vi "Set Tray Icon (file).vi"(0 "NotifyIcon in":refnum<class "NotifyIcon.lvclass">, 7 "Image file":path, 11 "error in (no error)":errorcluster) -> (4 "NotifyIcon out":refnum<class "NotifyIcon.lvclass">, 15 "error out":errorcluster)   [LabVIEW 2016, in "NotifyIcon.lvclass"]
doc: "This VI is used to set the icon that is associated with the context menu and shown in the notification area.\nThis VI loads a specified BMP, GIF, JPG, PNG, TIFF or ICO file and uses the content as the icon. The loaded file image is automatically resized to fit the notification area.\n\n\nStinus Olsen\nCIM Industrial Systems A/S\n22. Feb. 2011 15:06\nmailto: seo@cim.as"
uses:
  NotifyIcon.lvclass
  System.Drawing
panel:
  # "This VI belongs to the NotifyIcon Toolset. \nA toolset that makes it easy to create, control and manipulate a notification icon in the notification area of the Windows taskbar.\nThe toolset requires Microsoft .NET framework 2.0\n\n\nNOTICE -- YOU MUST LEAVE THIS NOTICE IN PLACE.  PER THE TERMS OF THE LICENSE BELOW, YOU MAY SUBLICENSE THIS SOFTWARE \nIN ANY WAY THAT DOES NOT CONFLICT WITH THIS LICENSE.\n\n### BSD License (http://www.opensource.org/licenses/bsd-license.php) Begin ###\n \nCopyright (c) 2011, Stinus Olsen <seo@cim.as>\n\nAll rights reserved.\n\nRedistribution and use in source and binary forms, with or without modification, are permitted provided that the following conditions are met:\n\n    * Redistributions of source code must retain the above copyright notice, this list of conditions and the following disclaimer.\n    * Redistributions in binary form must reproduce the above copyright notice, this list of conditions and the following disclaimer in the \n       documentation and/or other materials provided with the distribution.\n    * Neither the name of CIM Industrial Systems nor the names of its contributors may be used to endorse or promote products derived \n       from this software without specific prior written permission.\n\nTHIS SOFTWARE IS PROVIDED BY THE COPYRIGHT HOLDERS AND CONTRIBUTORS \"AS IS\" AND ANY EXPRESS OR IMPLIED WARRANTIES, \nINCLUDING, BUT NOT LIMITED TO, THE IMPLIED WARRANTIES OF MERCHANTABILITY AND FITNESS FOR A PARTICULAR PURPOSE ARE \nDISCLAIMED. IN NO EVENT SHALL THE COPYRIGHT OWNER OR CONTRIBUTORS BE LIABLE FOR ANY DIRECT, INDIRECT, INCIDENTAL,\n SPECIAL, EXEMPLARY, OR CONSEQUENTIAL DAMAGES (INCLUDING, BUT NOT LIMITED TO, PROCUREMENT OF SUBSTITUTE GOODS OR \nSERVICES; LOSS OF USE, DATA, OR PROFITS; OR BUSINESS INTERRUPTION) HOWEVER CAUSED AND ON ANY THEORY OF LIABILITY, \nWHETHER IN CONTRACT, STRICT LIABILITY, OR TORT (INCLUDING NEGLIGENCE OR OTHERWISE) ARISING IN ANY WAY OUT OF THE USE \nOF THIS SOFTWARE, EVEN IF ADVISED OF THE POSSIBILITY OF SUCH DAMAGE.\n\n### BSD License End ###"
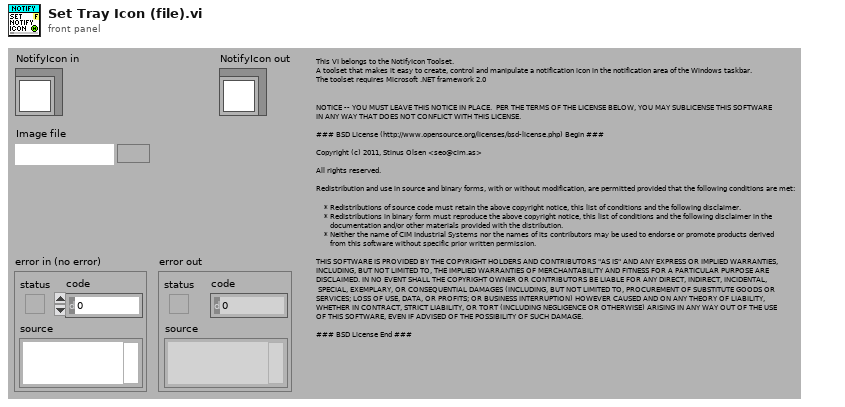
[diagram p1: front panel]
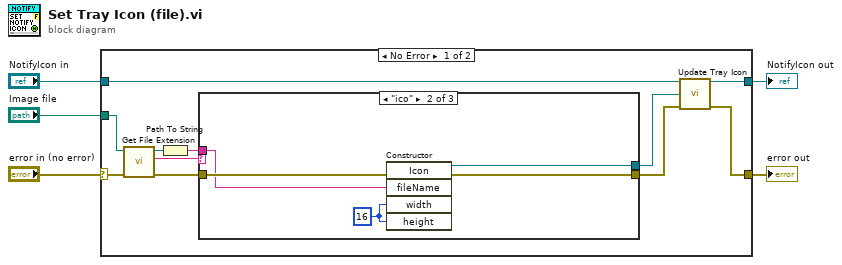
[diagram p0: block diagram]
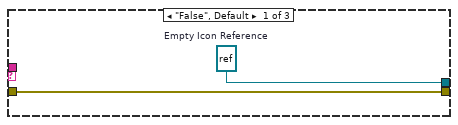
[diagram p2: hidden frame]
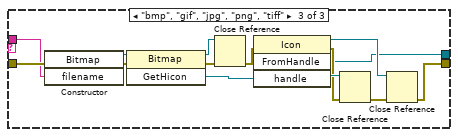
[diagram p3: hidden frame]
diagram:
  n1 = case shown="No Error" "error in (no error)" {
    selector: "error in (no error)" -> [w13 w38]
    tunnel: [w14 w38] -> w4
    tunnel: [w15 w37] -> w2
    tunnel: "NotifyIcon in" -> [w16 w37]
    tunnel: "Image file" -> [w11 _]
    frame No Error {
      n2 = call <vilib>:"Get File Extension.vi"("error in (no error)"=w13, "file"=w11) -> ("error out"=w12:errorcluster, "lowercase file extension"=w10:string, "dup file"=w7:path)  [unwired: 7 out]
      n3 = Path To String(path=w7) -> (string=w6:string)
      n4 = case shown="\"ico\"" w10 {
        tunnel: w12 -> [w18 w21 w27]
        tunnel: [w17 w22 w26] -> w8
        tunnel: [w18 w20 w24] -> w9
        tunnel: w6 -> [_ w19 w25]
        frame "False", Default {
          w17 = refnum<k24> refnum  # Empty Icon Reference
        }
        frame "ico" {
          w23 = 16 ("Int32 width")
          n5 = constructor class="Icon"(error in=w21, "fileName"=w19, "width"=w23, "height"=w23) -> (reference out=w22:refnum<k24>, error out=w20:errorcluster)  [unwired: 2 in, 4 out]
        }
        frame "bmp", "gif", "jpg", "png", "tiff" {
          n6 = constructor class="Bitmap"(error in=w27, "filename"=w25) -> (reference out=w36:refnum<k24>, error out=w35:errorcluster)  [unwired: 2 in, 2 out]
          n7 = invoke class="Bitmap" method="GetHicon"(reference=w36, error in=w35) -> (reference out=w31:refnum<k24>, error out=w32:errorcluster, "GetHicon"=w34:refnum<k24>)  [unwired: 1 in]
          n8 = Close Reference(reference=w31, error in (no error)=w32) -> (error out=w30:errorcluster)
          n9 = invoke class="Icon" method="FromHandle"(error in=w30, "handle"=w34) -> (reference out=w28:refnum<k24>, error out=w33:errorcluster, "FromHandle"=w26:refnum<k24>)  [unwired: 2 in, 1 out]
          n10 = Close Reference(reference=w34, error in (no error)=w33) -> (error out=w29:errorcluster)
          n11 = Close Reference(reference=w28, error in (no error)=w29) -> (error out=w24:errorcluster)
        }
      }
      n12 = call "Update Tray Icon.vi"("NotifyIcon in"=w16, "Icon Reference"=w8, "error in (no error)"=w9) -> ("NotifyIcon out"=w15:refnum<class "NotifyIcon.lvclass">, "error out"=w14:errorcluster)  [unwired: 1 in, 10 out]
    }
    frame Error {
    }
  }
  "error out" <- w4
  "NotifyIcon out" <- w2
